vi "Monitor ConstantSet (Relay).vi"(8 "error in (no error)":errorcluster, 10 "Address (0)":i32, 11 "VISA resource name":refnum<visa-resource-name>) -> (0 "error out":errorcluster, 2 "RELAY":T1, 3 "VISA resource name out":refnum<visa-resource-name>)   [LabVIEW 2021, in "Environment Chamber.lvlib" / "Climatic Chamber.lvlib"]
doc: "<b>Constant monitor\n(P-200, P-300 controllers only)</B>\n\nReturns the time signal set point in constant setup (No.1)."
uses:
  Climatic Chamber.lvlib
  Private/Type Defs/TimeSig ConstSetting Cluster.ctl
  Private/Type Defs/Constant OptionParameter Enum.ctl
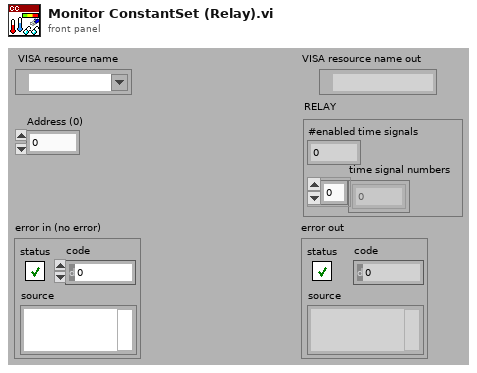
[diagram p1: front panel]
types:
  T1 = typedef "Environment Chamber.lvlib/Climatic Chamber.lvlib/TimeSig ConstSetting Cluster.ctl" = cluster{"#enabled time signals":i32, "time signal numbers":i32[]}
  T2 = typedef "Environment Chamber.lvlib/Climatic Chamber.lvlib/Constant OptionParameter Enum.ctl" = enum16{"TEMP", "HUMI", "REF", "RELAY", "PTC"}
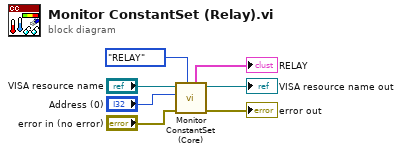
[diagram p0: block diagram]
diagram:
  n1 = call "Monitor ConstantSet (Core).vi"("Setpoint (TEMP)"=Constant_OptionParameter_Enum."RELAY", "error in (no error)"="error in (no error)", "Address (0)"="Address (0)", "VISA resource name"="VISA resource name") -> ("error out"=→"error out":errorcluster, "VISA resource name out"=→"VISA resource name out":refnum<visa-resource-name>, "RELAY"=→"RELAY":T1)  [unwired: 2 in, 3 out]
